vi "Fit ASCII Peak.vi"() -> ()   [LabVIEW 2016]
uses:
  <vilib>/Utility/file.llb/Read Delimited Spreadsheet (DBL).vi
  Smooth Background DBL.vi
  <vilib>/Analysis/NI_AALPro.lvlib
panel:
  out "Fit":T1(array[cluster])
  in  "Repeat":i32
  in  "Guess":T1(array[cluster])
  in  "Window end":dbl=697.0
  in  "Window start":dbl=690.0
  in  "Filter background":bool=TRUE
  out "Result":T2
  out "error":i32
  out "XY Graph":cluster{"all rows":dbl[], "Data out":dbl[]}[](graph)
  in  "File Path Control":path
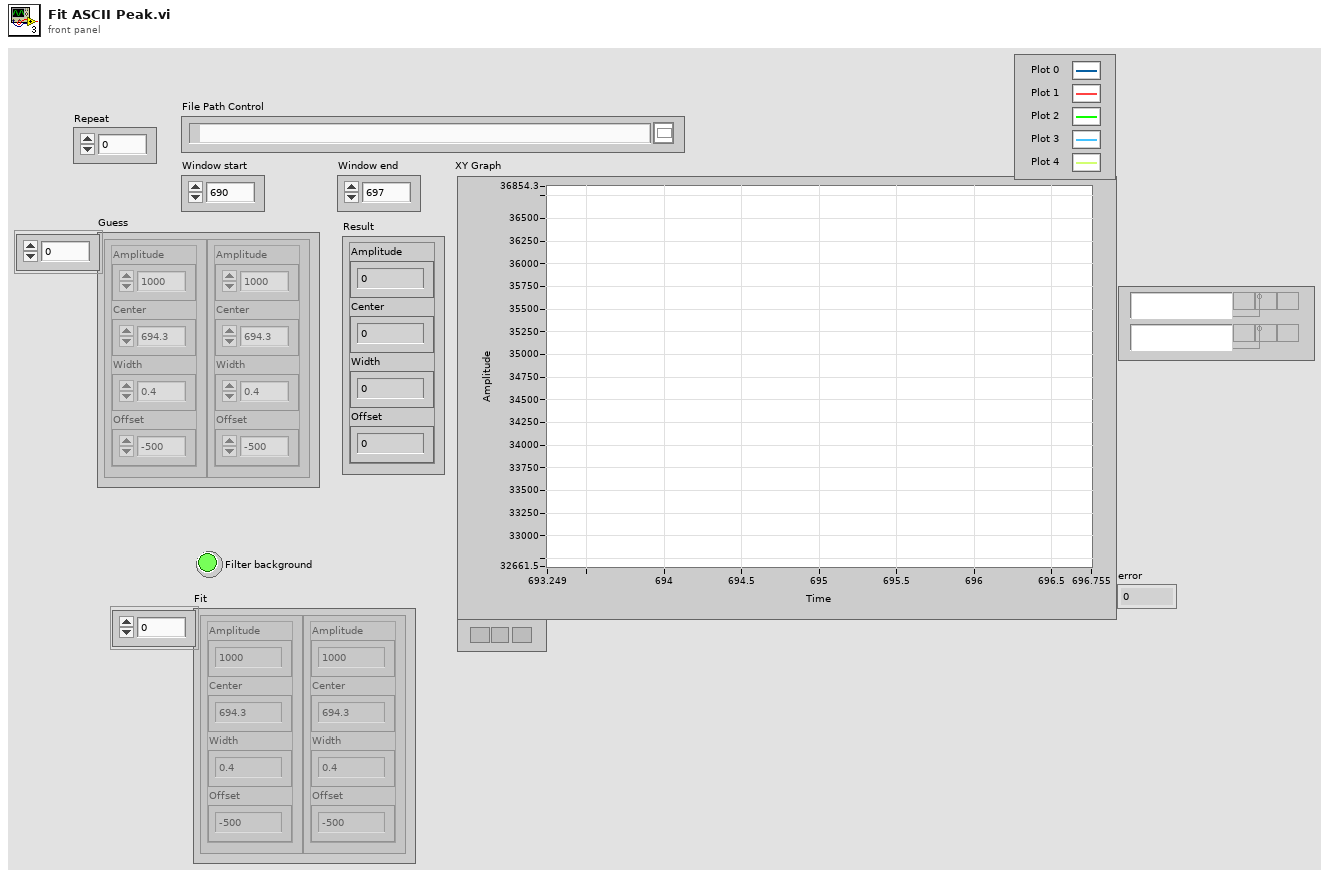
[diagram p1: front panel]
types:
  T1 = cluster{"Amplitude":dbl, "Center":dbl, "Width":dbl, "Offset":dbl}[]
  T2 = cluster{"Amplitude":dbl, "Center":dbl, "Width":dbl, "Offset":dbl}
  T3 = cluster{"amp min":dbl, "amp max":dbl, "center min":dbl, "center max":dbl, "deviation min":dbl, "deviation max":dbl, "offset min":dbl, "offset max":dbl}
  T4 = enum16{"Lowpass", "Highpass", "Bandpass", "Bandstop"}
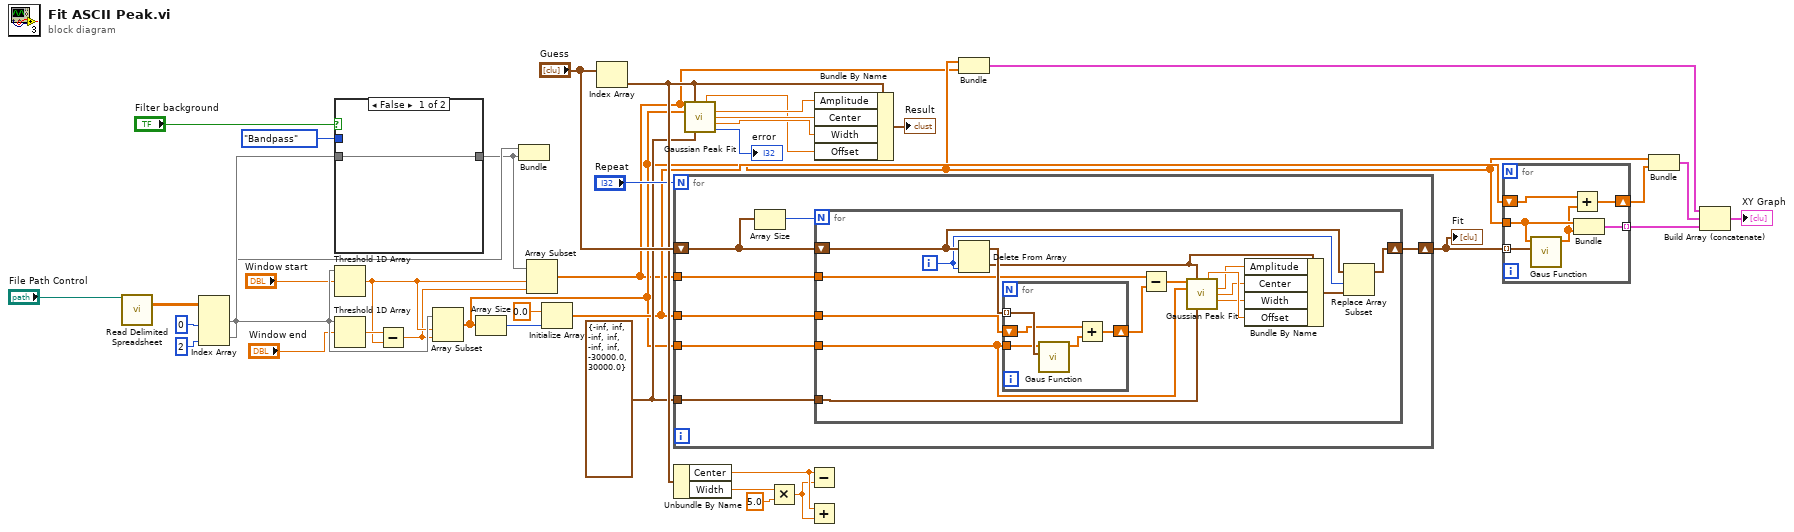
[diagram p0: block diagram]
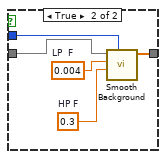
[diagram p2: hidden frame]
diagram:
  w8 = T3 {"amp min"=-inf, "amp max"=inf, "center min"=-inf, "center max"=inf, "deviation min"=-inf, "deviation max"=inf, "offset min"=-30000.0, "offset max"=30000.0} ("parameter bounds")
  n1 = call-poly <vilib>:"Read Delimited Spreadsheet.vi"("file path (dialog if empty)"="File Path Control") -> ("all rows"=w38:dbl[][])  [unwired: 9 in, 5 out]
  n2 = Index Array(array=w38, index (col) #1=0 ("disabled index (col)"), index (col) #2=2 ("index (col)")) -> (element #1=w30:dbl[], element #2=w32:dbl[])  [unwired: 2 in]
  n3 = case shown="False" "Filter background" {
    tunnel: T4."Bandpass" ("Type") -> [_ w45]
    tunnel: w32 -> [w40 w42]
    tunnel: [w40 w41] -> w26
    frame False {
    }
    frame True {
      w43 = 0.3  # HP F
      w44 = 0.004  # LP  F
      n4 = call-poly "Smooth Background.vi"("Type"=w45, "HP F"=w43, "LP  F"=w44, "Data"=w42) -> ("Data out"=w41:dbl[])  [unwired: 6 in, 1 out]
    }
  }
  n5 = Threshold 1D Array(2:"Window start", 3:w30) -> (0:w28:dbl)  [unwired: 1 in]
  n6 = Threshold 1D Array(2:"Window end", 3:w30) -> (0:w29:dbl)  [unwired: 1 in]
  n7 = Subtract(x=w29, y=w28) -> (x-y=w27:dbl)
  n8 = Array Subset(array=w30, index=w28, length=w27) -> (w3:dbl[])
  n9 = Array Size(array=w3) -> (size(s)=w11:i32)
  n10 = Bundle("all rows"=w30, "Data out"=w26) -> ()  [unwired: 1 in, 1 out]
  n11 = Array Subset(array=w26, index=w28, length=w27) -> (w1:dbl[])
  n12 = Initialize Array(0.0 ("element"), w11) -> (w5:dbl[])
  n13 = Index Array(array="Guess") -> (element=w13:T2)  [unwired: 1 in]
  n14 = for {
    N: "Repeat" -> [_]
    shift-right: [w47] -> w7
    shift-left: "Guess" -> [w51]
    tunnel: w3 -> [w52]
    tunnel: w5 -> [w49]
    tunnel: w1 -> [w48]
    tunnel: w8 -> [w46]
    n15 = Array Size(array=w51) -> (size(s)=w50:i32)
    n16 = for {
      N: w50 -> [_]
      tunnel: w52 -> [w53]
      tunnel: w49 -> [w67]
      tunnel: w48 -> [w65]
      shift-right: [w55] -> w47
      shift-left: w51 -> [w63]
      tunnel: w46 -> [w54]
      i -> [w56]
      n17 = Delete From Array(array=w63, index=w56) -> (deleted portion=w62:T2, array with subset deleted=w68:T1)  [unwired: 1 in]
      n18 = for {
        tunnel: w68 -> [w73] mode=indexing
        tunnel: w53 -> [w72]
        shift-right: [w69] -> w66
        shift-left: w67 -> [w71]
        n19 = call "Gaus Function.vi"("Fit params"=w73, "X"=w72) -> ("Y"=w70:dbl[])  [unwired: 9 in]
        n20 = Add(x=w71, y=w70) -> (x+y=w69:dbl[])
      }
      n21 = Subtract(x=w65, y=w66) -> (x-y=w64:dbl[])
      n22 = call <vilib>:"Gaussian Peak Fit.vi"("Y"=w64, "initial guess"=w62, "X"=w53, "parameter bounds"=w54) -> ("offset"=w61:dbl, "amplitude"=w60:dbl, "center"=w59:dbl, "standard deviation"=w58:dbl)  [unwired: 5 in, 3 out]
      n23 = Bundle By Name(cluster=w62, "Amplitude"=w60, "Center"=w59, "Width"=w58, "Offset"=w61) -> (w57:T2)
      n24 = Replace Array Subset(array=w63, new element=w57, index=w56) -> (w55:T1)
    }
  }
  "Fit" <- w7
  n25 = Unbundle By Name(w13) -> ("Center"=w24:dbl, "Width"=w25:dbl)
  n26 = call <vilib>:"Gaussian Peak Fit.vi"("Y"=w1, "initial guess"=w13, "X"=w3, "parameter bounds"=w8) -> ("offset"=w18:dbl, "amplitude"=w21:dbl, "center"=w20:dbl, "standard deviation"=w19:dbl, "error"=→"error":i32)  [unwired: 5 in, 2 out]
  n27 = Multiply(x=w25, y=5.0) -> (x*y=w22:dbl)
  n28 = Subtract(x=w24, y=w22) -> ()  [unwired: 1 out]
  n29 = Add(x=w24, y=w22) -> ()  [unwired: 1 out]
  n30 = Bundle By Name(cluster=w13, "Amplitude"=w21, "Center"=w20, "Width"=w19, "Offset"=w18) -> (→"Result":T2)
  n31 = Bundle(w3, w1) -> (w33:cluster{dbl[], dbl[]})  [unwired: 1 in]
  n32 = for {
    tunnel: [w79] -> w6 mode=indexing
    tunnel: w3 -> [w78]
    tunnel: w7 -> [w77] mode=indexing
    shift-right: [w74] -> w4
    shift-left: w5 -> [w76]
    n33 = call "Gaus Function.vi"("Fit params"=w77, "X"=w78) -> ("Y"=w75:dbl[])  [unwired: 9 in]
    n34 = Add(x=w76, y=w75) -> (x+y=w74:dbl[])
    n35 = Bundle(w78, "Y"=w75) -> (w79:cluster{dbl[], "Y":dbl[]})  [unwired: 1 in]
  }
  n36 = Bundle(w3, w4) -> (w2:cluster{dbl[], dbl[]})  [unwired: 1 in]
  n37 = Build Array (concatenate)(w33, w2, w6) -> (→"XY Graph":cluster{dbl[], "Y":dbl[]}[])
